vi "En-queue RT data element.vi"(8 "Data":variant, 9 "Message":string, 11 "RT Queues":T1) -> (0 "error out":errorcluster, 1 "timed out?":bool, 3 "RT Queues out":T1)   [LabVIEW 2018]
uses:
  Type Defs/Queues cluster.ctl
  Chris VIs/Message Scheduler/message scheduler.lvclass
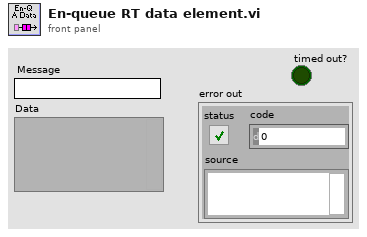
[diagram p1: front panel]
types:
  T1 = typedef "Queues cluster.ctl" = cluster{"RT Message":refnum<queue>, "RT Comms":refnum<queue>, "RT Data":refnum<queue>, "RT FIFO":refnum<queue>, "message scheduler":refnum<class "message scheduler.lvclass">}
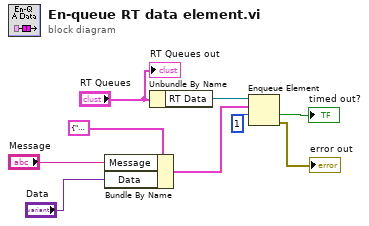
[diagram p0: block diagram]
diagram:
  n1 = Bundle By Name(cluster=cluster{"Message":string, "Data":variant} {"Message"="", "Data"=variant} ("element"), "Message"="Message", "Data"="Data") -> (w4:cluster{"Message":string, "Data":variant})
  n2 = Unbundle By Name("RT Queues") -> ("RT Data"=w8:refnum<queue>)
  n3 = Enqueue Element(queue=w8, element=w4, timeout in ms (-1)=1) -> (timed out?=→"timed out?":bool, error out=→"error out":errorcluster)  [unwired: 1 in, 1 out]
  "RT Queues out" <- "RT Queues"
